vi "Acquisition_c.vi"() -> (4 "Acquired_Data":dbl(graph))   [LabVIEW 2023]
doc: "This VI acquire data that were generated be the Generator VI.\nTransfer of thet data happens under Queue LV2."
uses:
  Controls/Operation_Queue.ctl
panel:
  out "Error_Out":errorcluster
  in  "Error_In":errorcluster
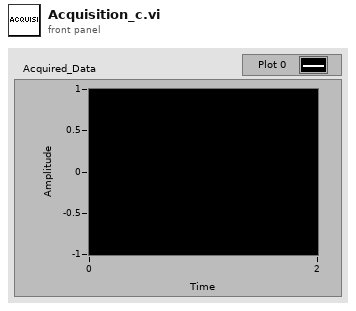
[diagram p1: front panel]
types:
  T1 = typedef "Operation_Queue.ctl" = enum16{"Initialize", "Enqueue", "Dequeue", "Sum"}
  T2 = enum16{"Left Button", "Center Button", "Right Button", "Window Close"}
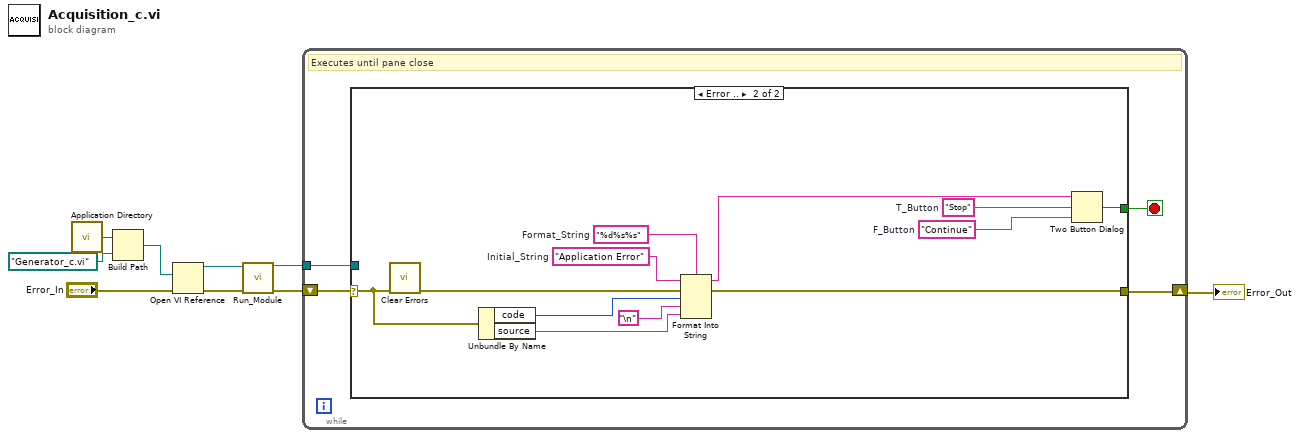
[diagram p0: block diagram]
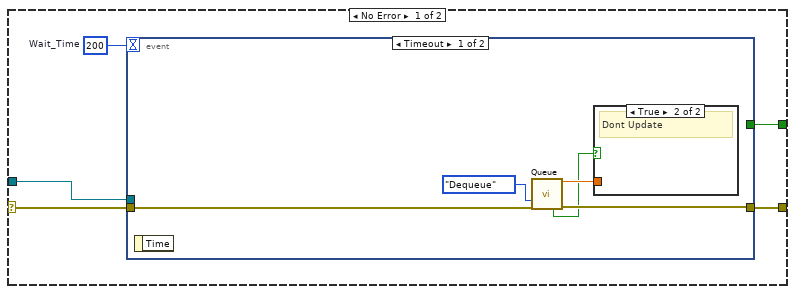
[diagram p2: hidden frame]
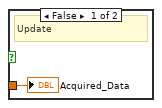
[diagram p3: hidden frame]
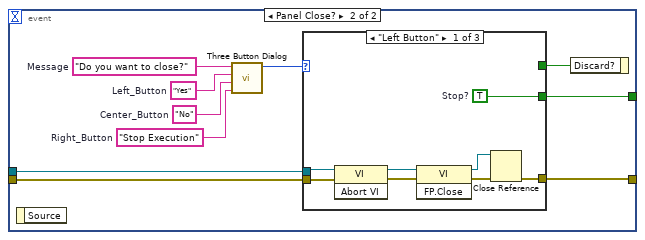
[diagram p4: hidden frame]
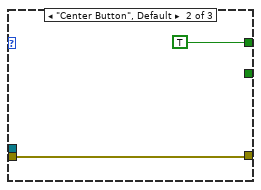
[diagram p5: hidden frame]
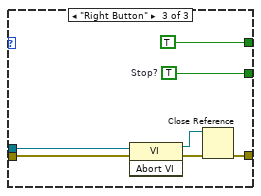
[diagram p6: hidden frame]
diagram:
  n1 = call <vilib>:"Application Directory.vi"() -> ("Application Directory"=w7:path)
  n2 = Build Path(base path=w7, name or relative path=path "Generator_c.vi") -> (appended path=w8:path)
  n3 = Open VI Reference(vi path=w8, error in (no error)="Error_In") -> (vi reference=w2:refnum<vi>, error out=w4:errorcluster)  [unwired: 4 in]
  n4 = call "Run_Module.vi"("VI_In"=w2, "Error_In"=w4) -> ("VI_Out"=w3:refnum<vi>, "Error_Out"=w1:errorcluster)  [unwired: 12 in]
  n5 = while {
    tunnel: w3 -> [w10]
    shift-right: [w11] -> w5
    shift-left: w1 -> [w12]
    stop <- w13 stop-if-true
    # "Executes until pane close"
    n6 = case shown="Error .." w12 {
      selector: w12 -> [w16 w57]
      tunnel: [w17 w52] -> w13
      tunnel: [w15 w55] -> w11
      tunnel: w10 -> [w14 _]
      frame No Error {
        w18 = 200  # Wait_Time
        n7 = event shown="[0] Timeout" {
          selector: _ -> [_ _]
          dyn-events: _ -> [_ _]
          timeout: w18 -> [_ _]
          tunnel: [_ w28] -> w17
          tunnel: w16 -> [w23 w26]
          tunnel: [w22 w27] -> w15
          tunnel: w14 -> [_ w25]
          event Timeout {
            n8 = event-data() -> ()  [unwired: 1 in, 1 out]
            n9 = call "Queue.vi"("Operation"=Operation_Queue."Dequeue" ("Operation_Queue"), "Error_In"=w23) -> ("Element_Out"=w20:dbl, "Underflow"=w19:bool, "Error_Out"=w22:errorcluster)  [unwired: 9 in, 2 out]
            n10 = case shown="True" w19 {
              tunnel: w20 -> [w24 _]
              frame False {
                # "Update"
                "Acquired_Data" <- w24
              }
              frame True {
                # "Dont Update"
              }
            }
          }
          event Panel Close? {
            w31 = "Stop Execution"  # Right_Button
            w32 = "No"  # Center_Button
            w33 = "Yes"  # Left_Button
            w34 = "Do you want to close?"  # Message
            n11 = event-data() -> ()  [unwired: 1 in, 1 out]
            n12 = call <vilib>:"Three Button Dialog.vi"("Right Button Text (\"Cancel\")"=w31, "Center Button Text (\"No\")"=w32, "Left Button Text (\"Yes\")"=w33, "message"=w34) -> ("Which Button?"=w30:T2)  [unwired: 7 in]
            n13 = case shown="\"Left Button\"" w30 {
              tunnel: [_ TRUE ("Discard?") TRUE ("Discard?")] -> w29
              tunnel: [w42 _ w51] -> w28
              tunnel: [w39 w43 w47] -> w27
              tunnel: w26 -> [w36 w43 w46]
              tunnel: w25 -> [w37 _ w45]
              frame "Left Button" {
                w42 = TRUE  # Stop?
                n14 = invoke class="VI" method="Abort VI"(reference=w37, error in=w36) -> (reference out=w38:refnum<vi>, error out=w35:errorcluster)  [unwired: 1 in, 1 out]
                n15 = invoke class="VI" method="FP.Close"(reference=w38, error in=w35) -> (reference out=w41:refnum<vi>, error out=w40:errorcluster)  [unwired: 1 in, 1 out]
                n16 = Close Reference(reference=w41, error in (no error)=w40) -> (error out=w39:errorcluster)
              }
              frame "Center Button", Default {
              }
              frame "Right Button" {
                w51 = TRUE  # Stop?
                n17 = invoke class="VI" method="Abort VI"(reference=w45, error in=w46) -> (reference out=w49:refnum<vi>, error out=w48:errorcluster)  [unwired: 1 in, 1 out]
                n18 = Close Reference(reference=w49, error in (no error)=w48) -> (error out=w47:errorcluster)
              }
            }
            n19 = event-data ("Event Filter Node")("Discard?"=w29) -> ()  [unwired: 1 in, 1 out]
          }
        }
      }
      frame Error {
        w59 = "%d%s%s"  # Format_String
        w60 = "Application Error"  # Initial_String
        w61 = "Stop"  # T_Button
        w62 = "Continue"  # F_Button
        n20 = call <vilib>:"Clear Errors.vi"("error in (no error)"=w57) -> ("error out"=w56:errorcluster)  [unwired: 5 in, 1 out]
        n21 = Unbundle By Name(w57) -> ("code"=w54:i32, "source"=w53:string)
        n22 = Format Into String(format string=w59, initial string=w60, error in=w56, w54, "\n", w53) -> (resulting string=w63:string, error out=w55:errorcluster)
        n23 = Two Button Dialog(message=w63, 1:w62, 2:w61) -> (T button?=w52:bool)
      }
    }
  }
  "Error_Out" <- w5
